vi "testFlattenPlaneAngleToXML.vi"() -> ()   [LabVIEW 2012, in "UnitsAndXML.lvlib"]
uses:
  <userlib>/Common/UnitsAndXML/UnitsAndXML.lvlib
  <userlib>/Common/UnitsAndXML/FlattenItemWithUnitToXML/FlattenPlaneAngleToXML/PlaneAngleUnit.ctl
  <userlib>/Common/UnitsAndXML/SupportFiles/Position/Position.lvclass
  <userlib>/Common/UnitsAndXML/FlattenItemWithUnitToXML/FlattenPlaneAngleToXML/typeMethods/flattenPlaneAngleToXML_Array.vi
  <userlib>/Common/UnitsAndXML/FlattenItemWithUnitToXML/FlattenPlaneAngleToXML/typeMethods/flattenPlaneAngleToXML_Scalar.vi
panel:
  out "error out":errorcluster
  out "xmlStringScalar 2":string
  out "xmlStringArray 2":string
  in  "PlaneAngleUnitInXML":T1
  out "xmlStringArray":string
  out "xmlStringScalar":string
  in  "angles":dbl[unit][](array[numeric])=[0.2617993877991494, 0.5235987755982988, 0.7853981633974483, 1.0471975511965976]
  in  "angle":dbl[unit]=0.2617993877991494
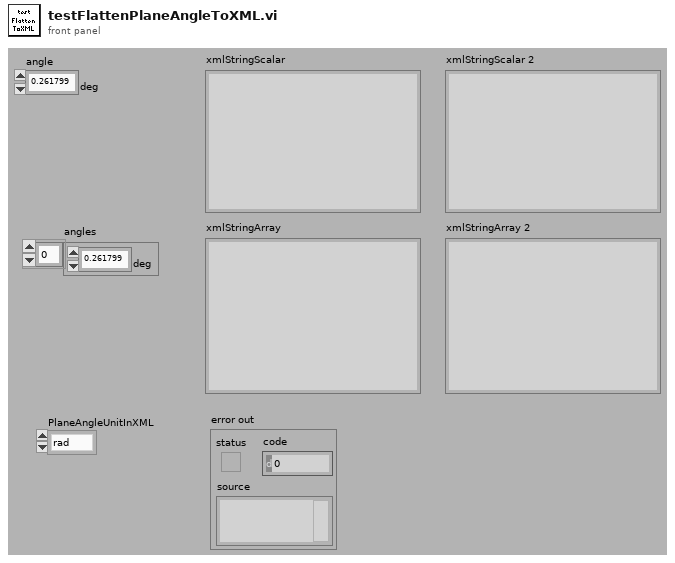
[diagram p1: front panel]
types:
  T1 = typedef "UnitsAndXML.lvlib/PlaneAngleUnit.ctl" = enum16{"rad", "deg", "'", "\""}
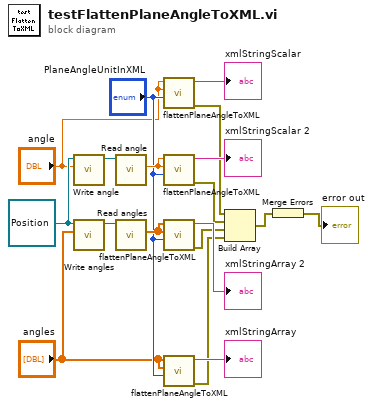
[diagram p0: block diagram]
diagram:
  w4 = refnum<class "Position.lvclass"> refnum ("Position in")
  n1 = call <userlib>:"Write angle.vi"("angle"="angle", "Position in"=w4) -> ("Position out"=w13:refnum<class "Position.lvclass">)  [unwired: 8 in, 1 out]
  n2 = call <userlib>:"Write angles.vi"("angles"="angles", "Position in"=w4) -> ("Position out"=w14:refnum<class "Position.lvclass">)  [unwired: 8 in, 1 out]
  n3 = call <userlib>:"Read angle.vi"("Position in"=w13) -> ("angle"=w12:dbl[unit])  [unwired: 8 in, 2 out]
  n4 = call <userlib>:"Read angles.vi"("Position in"=w14) -> ("angles"=w11:dbl[unit][])  [unwired: 8 in, 2 out]
  n5 = call-poly <userlib>:"flattenPlaneAngleToXML.vi"("planeAngleUnitInXML"="PlaneAngleUnitInXML", "planeAngleAgain"="angle", "planeAngle"="angle") -> ("error out"=w9:errorcluster, "xmlString"=→"xmlStringScalar":string)  [unwired: 7 in]
  n6 = call-poly <userlib>:"flattenPlaneAngleToXML.vi"("planeAngleUnitInXML"="PlaneAngleUnitInXML", "planeAngleAgain"=w12, "planeAngle"=w12) -> ("error out"=w8:errorcluster, "xmlString"=→"xmlStringScalar 2":string)  [unwired: 7 in]
  n7 = call-poly <userlib>:"flattenPlaneAngleToXML.vi"("planeAngleUnitInXML"="PlaneAngleUnitInXML", "planeAngleAgain"=w11, "planeAngle"=w11) -> ("error out"=w7:errorcluster, "xmlString"=→"xmlStringArray 2":string)  [unwired: 7 in]
  n8 = call-poly <userlib>:"flattenPlaneAngleToXML.vi"("planeAngleUnitInXML"="PlaneAngleUnitInXML", "planeAngleAgain"="angles", "planeAngle"="angles") -> ("error out"=w6:errorcluster, "xmlString"=→"xmlStringArray":string)  [unwired: 7 in]
  n9 = Build Array(w9, w8, w7, w6) -> (w10:errorcluster[])
  n10 = Merge Errors(w10) -> (→"error out":errorcluster)
